vi "Test Get Connected Entities.vi"() -> ()   [LabVIEW 2014]
uses:
  types/Entities.ctl
panel:
  out "Count of constant at top level in VI":i32
  out "Wired Terminal Label":string
  out "Wired Terminal Class Name":string
  out "Count of wire terminals at top level in VI":i32
  in  "vi path":path=path "C:/Users/lubo/Documents/LabView/LabVIEW-Universal-Transcriptor/Test/Example Terminals 1.vi"
  # "This example is supposed to run on\n\"Example Terminals 1.vi\""
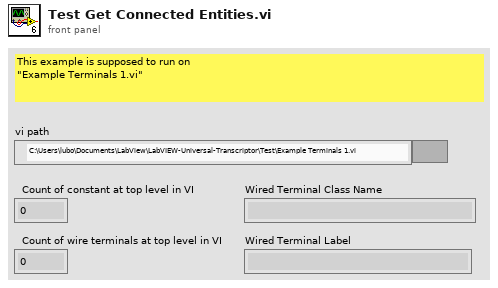
[diagram p1: front panel]
types:
  T1 = typedef "Entities.ctl" = string
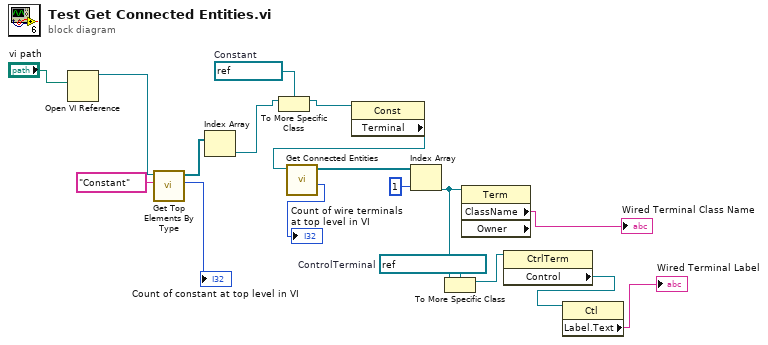
[diagram p0: block diagram]
diagram:
  w7 = refnum<vi> refnum  # ControlTerminal
  w14 = refnum<vi> refnum  # Constant
  n1 = Open VI Reference(vi path="vi path") -> (vi reference=w17:refnum<vi>)  [unwired: 5 in, 1 out]
  n2 = call "Get Top Elements By Type.vi"("type"=T1 "Constant", "VI in"=w17) -> ("# of Refs"=→"Count of constant at top level in VI":i32, "References"=w16:refnum<vi>[])  [unwired: 7 in, 1 out]
  n3 = Index Array(array=w16) -> (element=w15:refnum<vi>)  [unwired: 1 in]
  n4 = To More Specific Class(target class=w14, reference=w15) -> (specific class reference=w13:refnum<vi>)  [unwired: 1 in, 1 out]
  n5 = property class="Const"(reference=w13) -> ("Terminal"=w12:refnum<vi>)  [unwired: 1 in, 2 out]
  n6 = call "Get Connected Entities.vi"("terminal ref."=w12) -> ("#terminals"=→"Count of wire terminals at top level in VI":i32, "Connected Wire.Terminals[]"=w10:refnum<vi>[])  [unwired: 9 in]
  n7 = Index Array(array=w10, index=1) -> (element=w5:refnum<vi>)
  n8 = To More Specific Class(target class=w7, reference=w5) -> (specific class reference=w6:refnum<vi>)  [unwired: 1 in, 1 out]
  n9 = property class="Term" props=["ClassName", "Owner"](reference=w5) -> ("ClassName"=→"Wired Terminal Class Name":string)  [unwired: 1 in, 3 out]
  n10 = property class="CtrlTerm"(reference=w6) -> ("Control"=w4:refnum<vi>)  [unwired: 1 in, 2 out]
  n11 = property class="Ctl"(reference=w4) -> ("Label.Text"=→"Wired Terminal Label":string)  [unwired: 1 in, 2 out]
